vi "Tree - Select Row.vi"(8 "error in (no error)":errorcluster, 9 "Active Cell:String":string, 10 "Color Box":u32(colorbox), 11 "TreeControl in":refnum<vi>) -> (0 "error out":errorcluster, 3 "TreeControl out":refnum<vi>)   [LabVIEW 2020]
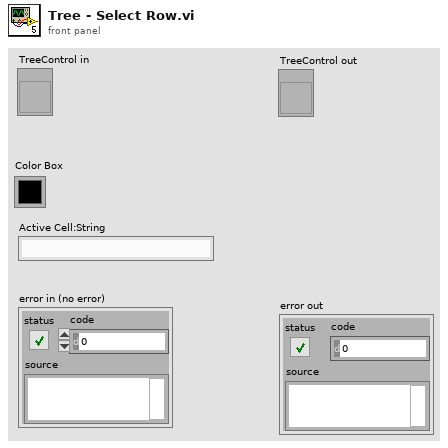
[diagram p1: front panel]
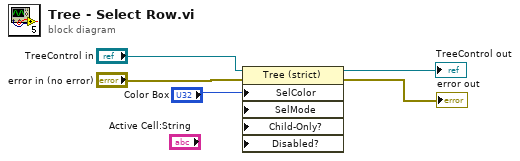
[diagram p0: block diagram]
diagram:
  n1 = property class="Tree (strict)" props=["SelColor", "SelMode", "Child-Only?", "Disabled?"](reference="TreeControl in", error in="error in (no error)", "SelColor"="Color Box") -> (reference out=→"TreeControl out":refnum<vi>, error out=→"error out":errorcluster)  [unwired: 3 in]
